vi "Objective Align - Crop Image.vi"(0 "Image Ref":T1, 5 "ROI Size":i32, 7 "Pixel Size (µm)":dbl, 9 "XY Step Size (µm)":dbl, 12 "Input Image - U16":u16[][](array[numeric])) -> (4 "Output Image Stack":u16[][][](array[numeric]), 8 "Coord":i32[][](array[numeric]))   [LabVIEW 2021]
uses:
  <vilib>/vision/Image Controls.llb/IMAQ Image.ctl
  Display Module/Display Module Custom Controls/ROI Descriptor.ctl
panel:
  out "full":u16[][](graph)
  out "ROI2":u16[][](graph)
  out "ROI1":u16[][](graph)
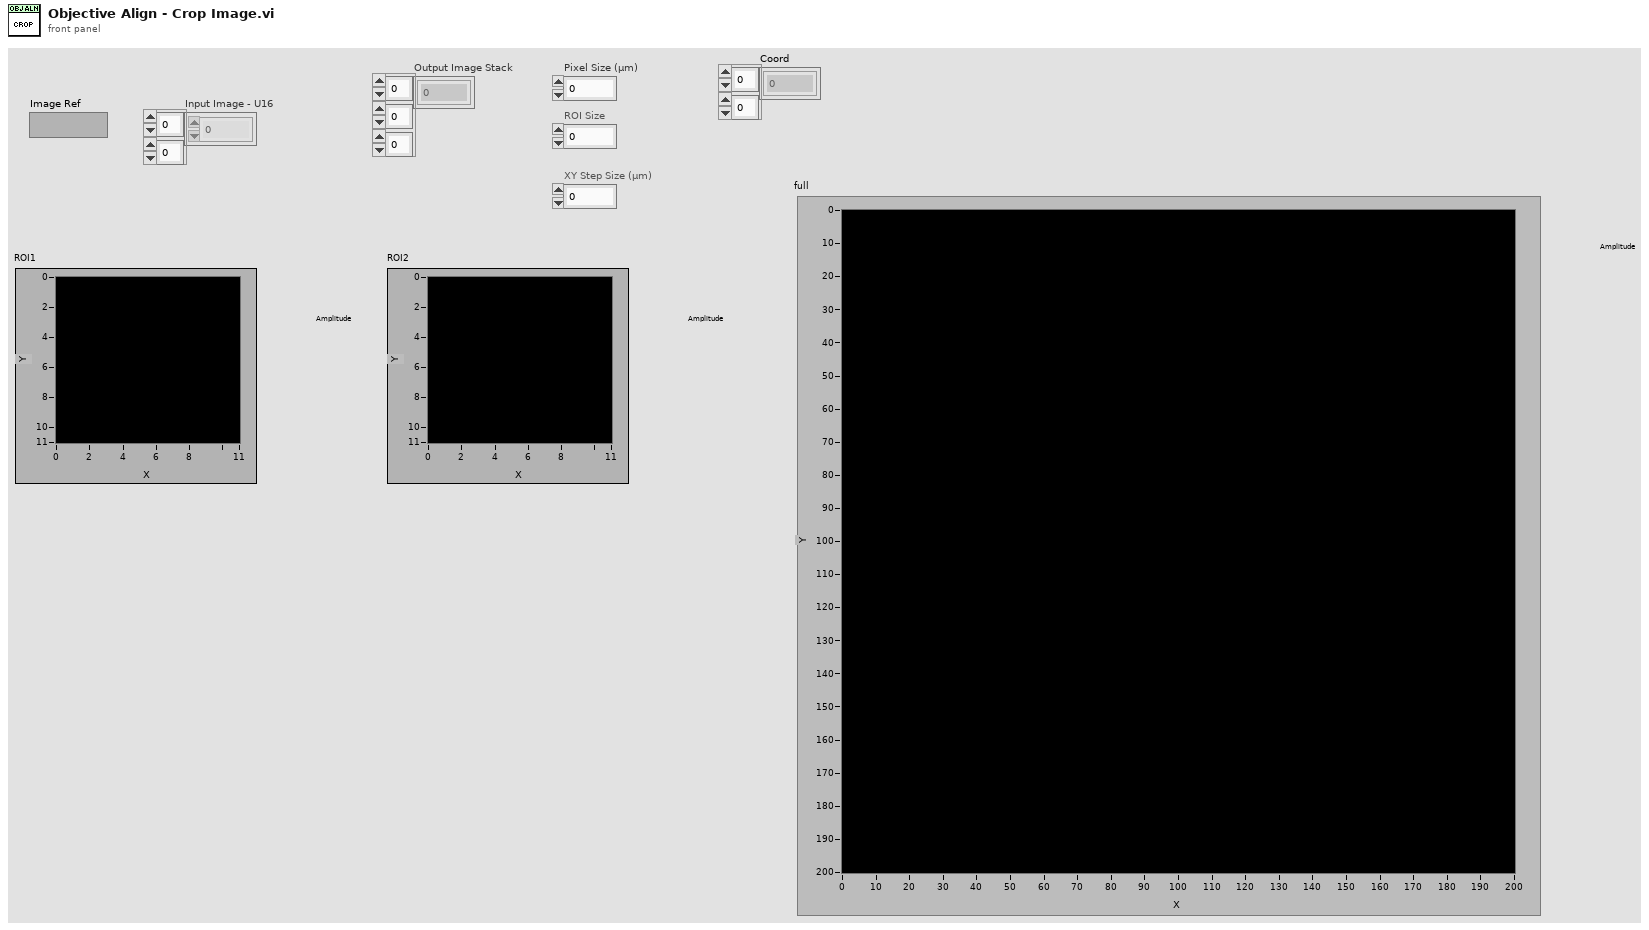
[diagram p1: front panel]
types:
  T1 = typedef "IMAQ Image.ctl" = refnum<image>
  T2 = typedef "ROI Descriptor.ctl" = cluster{"Global Rectangle":i32[], "Contours":cluster{"Contour Type":u32, "ROI Type":u32, "Points":i32[]}[]}
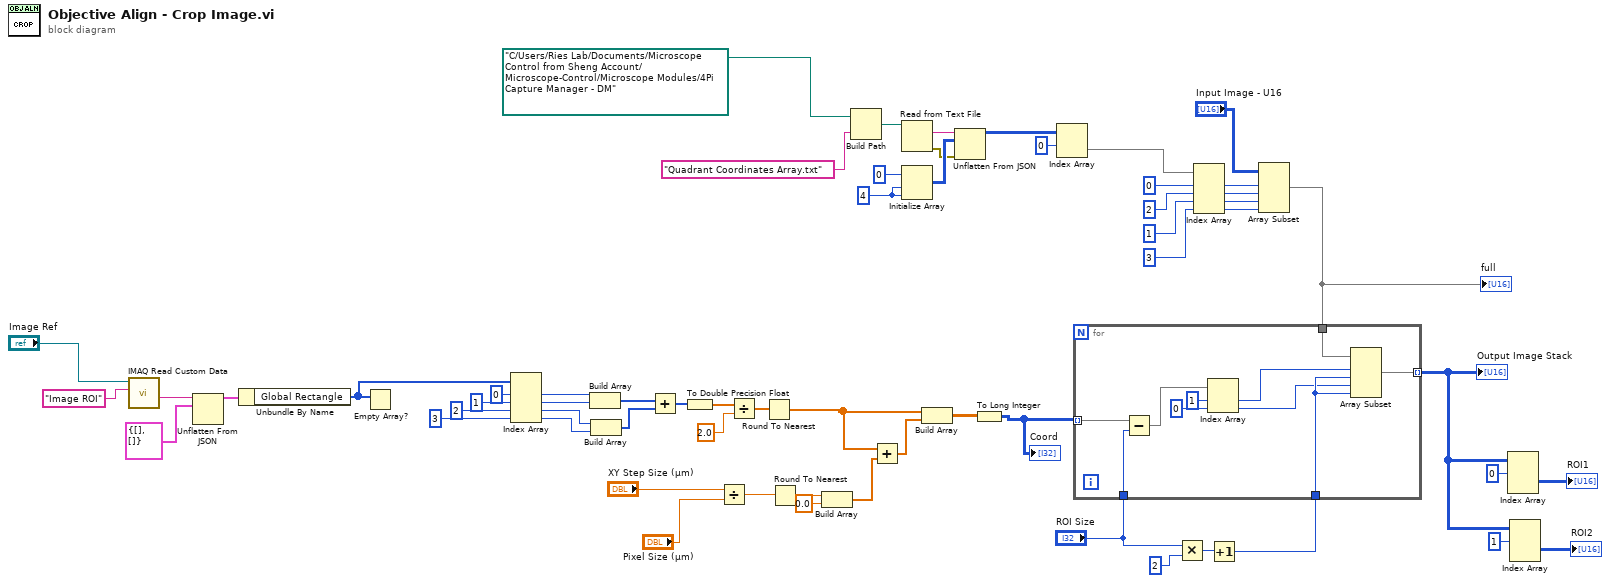
[diagram p0: block diagram]
diagram:
  w16 = 4 ("dimension size")
  n1 = call "IMAQ Read Custom Data"("Key"="Image ROI", "Image"="Image Ref") -> ("Custom Data Out"=w31:string)  [unwired: 7 in, 2 out]
  n2 = Unflatten From JSON(JSON string=w31, type and defaults=T2 {"Global Rectangle"=[], "Contours"=[]} ("Image ROI Descriptor")) -> (value=w33:T2)  [unwired: 5 in, 1 out]
  n3 = Unbundle By Name(w33) -> ("Global Rectangle"=w34:i32[])
  n4 = Empty Array?(array=w34) -> ()  [unwired: 1 out]
  n5 = Index Array(array=w34, index #1=0 ("index"), index #2=1 ("index"), index #3=2 ("index"), index #4=3 ("index")) -> (element #1=w47:i32, element #2=w48:i32, element #3=w49:i32, element #4=w50:i32)
  n6 = Build Array(w47, w48) -> (w51:i32[])
  n7 = Build Array(w49, w50) -> (w52:i32[])
  n8 = Add(x=w51, y=w52) -> (x+y=w45:i32[])
  n9 = To Double Precision Float(number=w45) -> (double precision float=w44:dbl[])
  n10 = Divide(x="XY Step Size (µm)", y="Pixel Size (µm)") -> (x/y=w56:dbl)
  n11 = Divide(x=w44, y=2.0) -> (x/y=w53:dbl[])
  n12 = Round To Nearest(number=w53) -> (nearest integer value=w1:dbl[])
  n13 = Round To Nearest(number=w56) -> (nearest integer value=w57:dbl)
  n14 = Build Array(w57, 0.0 ("element")) -> (w59:dbl[])
  n15 = Build Path(base path=path "C:/Users/Ries Lab/Documents/Microscope Control from Sheng Account/Microscope-Control/Microscope Modules/4Pi Capture Manager - DM" ("path"), name or relative path="Quadrant Coordinates Array.txt") -> (appended path=w19:path)
  n16 = Add(x=w1, y=w59) -> (x+y=w60:dbl[])
  n17 = Read from Text File(file (use dialog)=w19) -> (text=w18:string, error out=w17:errorcluster)  [unwired: 3 in, 2 out]
  n18 = Initialize Array(0 ("element"), w16, w16) -> (w20:i32[][])
  n19 = Build Array(w1, w60) -> (w24:dbl[][])
  n20 = Unflatten From JSON(JSON string=w18, type and defaults=w20, error in (no error)=w17) -> (value=w14:i32[][])  [unwired: 4 in, 1 out]
  n21 = To Long Integer(number=w24) -> (32bit integer=w23:i32[][])
  "Coord" <- w23
  n22 = Index Array(array=w14, index (row)=0) -> (element=w8:i32[])  [unwired: 1 in]
  n23 = Multiply(x="ROI Size", y=2) -> (x*y=w37:i32)
  n24 = Index Array(array=w8, index #1=0 ("index"), index #2=2 ("index"), index #3=1 ("index"), index #4=3 ("index")) -> (element #1=w6:i32, element #2=w5:i32, element #3=w4:i32, element #4=w3:i32)
  n25 = Increment(x=w37) -> (x+1=w38:i32)
  n26 = Array Subset(array="Input Image - U16", index (row)=w6, length (row)=w5, index (col)=w4, length (col)=w3) -> (w2:u16[][])
  "full" <- w2
  n27 = for {
    tunnel: w38 -> [w70]
    tunnel: "ROI Size" -> [w69]
    tunnel: w2 -> [w68]
    tunnel: [w62] -> w25 mode=indexing
    tunnel: w23 -> [w61] mode=indexing
    n28 = Subtract(x=w61, y=w69) -> (x-y=w67:i32[])
    n29 = Index Array(array=w67, index #1=1 ("index"), index #2=0 ("index")) -> (element #1=w64:i32, element #2=w63:i32)
    n30 = Array Subset(array=w68, index (row)=w64, length (row)=w70, index (col)=w63, length (col)=w70) -> (w62:u16[][])
  }
  "Output Image Stack" <- w25
  n31 = Index Array(array=w25, index (dim 0)=0 ("index (page)")) -> (element=→"ROI1":u16[][])  [unwired: 2 in]
  n32 = Index Array(array=w25, index (dim 0)=1 ("index (page)")) -> (element=→"ROI2":u16[][])  [unwired: 2 in]
